vi "Ch_setup_string.vi"(6 "Ch & spans":T1[](array[typedef]) {"low limit (-10V)" format="%.3f"; "high limit (10V)" format="%.3f"}) -> (1 "Output string":string)   [LabVIEW 2013]
uses:
  Controls/Ch_and_Spans.ctl
  Globals/Meas_global.vi
panel:
  out "length":i32
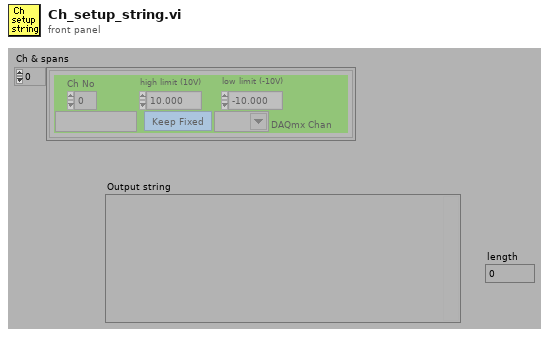
[diagram p1: front panel]
types:
  T1 = typedef "Ch_and_Spans.ctl" = cluster{"high limit (10V)":sgl, "low limit (-10V)":sgl, "Ch No":i16, "Var name":string, "Use Latest Calib":bool, "DAQmx Chan":tag}
  T2 = typedef "Analysis_info_cluster.ctl" = cluster{"Colour":u32, "Inst type":T3, "Inst name":string, "Symbol":string, "Code name":string, "Extra Info":string, "Inst Array":T4, "Extra Titles":string[], "Extra Values":string[], "U":dbl, "u^2":dbl, "u^3":dbl, "u^4":dbl, "Skew_u":dbl, "Kurt_u":dbl, "Sd Error in Mean":dbl, "% u'/U":dbl, "X":dbl, "Y":dbl, "Z":dbl, "Timescale integral to 25%":dbl, "Sd Error in Variance":dbl, "Calib File":path, "Calib Constants":dbl[], "Output Position":bool, "Full Stats":bool, "Av Sampling Rate":dbl, "Av No of Samples":dbl, "Total Meas Time (s)":dbl, "ADAM Ch Name":string}
  T3 = typedef "Inst_type.ctl" = enum16{"Propeller anemometer", "Raw voltage", "Pressure Transducer", "Pitot-static tube", "Preston tube", "Hot wire", "Cross wire 1", "Cross wire 2", "Generic Linear", "Generic Polynomial", "Generic BackPoly", "Fast FID", "Thermocouple", "Cold wire", "Pulsed Wire", "LDA Vel", "LDA Tran time", "LDA Arr time"}
  T4 = typedef "Instrument_Array.ctl" = enum16{"PWA", "LDA", "Analogue"}
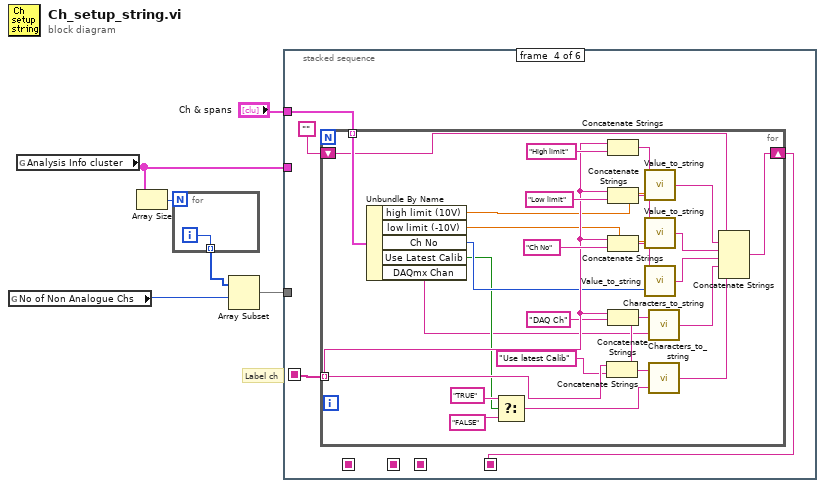
[diagram p0: block diagram]
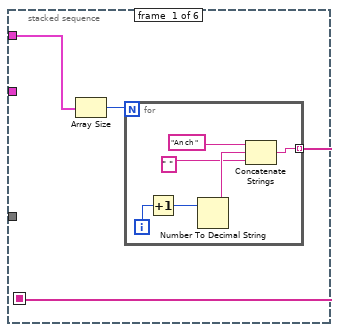
[diagram p2: hidden frame]
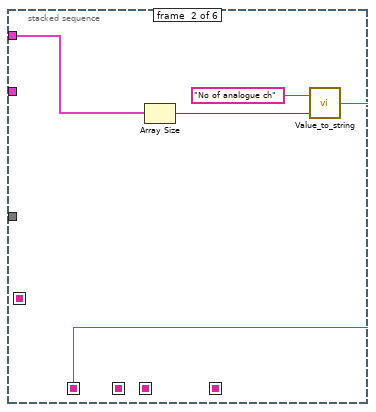
[diagram p3: hidden frame]
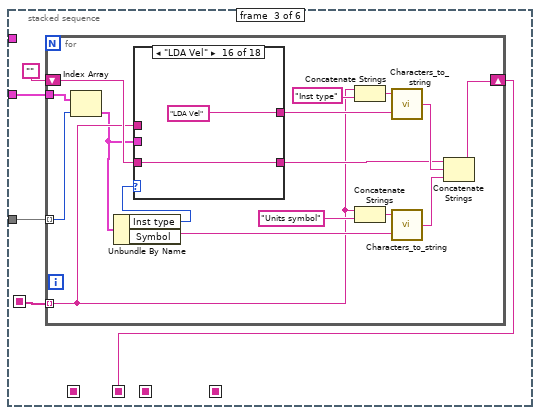
[diagram p4: hidden frame]
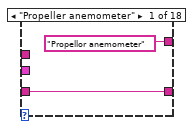
[diagram p5: hidden frame]
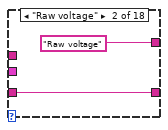
[diagram p6: hidden frame]
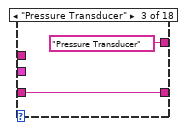
[diagram p7: hidden frame]
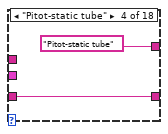
[diagram p8: hidden frame]
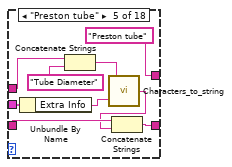
[diagram p9: hidden frame]
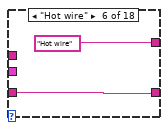
[diagram p10: hidden frame]
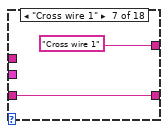
[diagram p11: hidden frame]
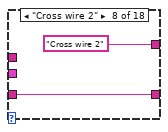
[diagram p12: hidden frame]
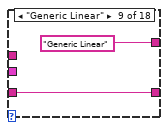
[diagram p13: hidden frame]
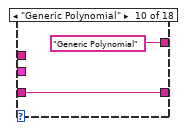
[diagram p14: hidden frame]
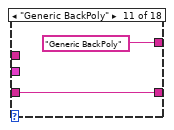
[diagram p15: hidden frame]
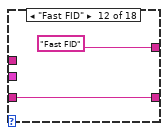
[diagram p16: hidden frame]
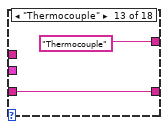
[diagram p17: hidden frame]
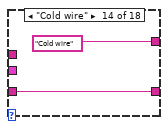
[diagram p18: hidden frame]
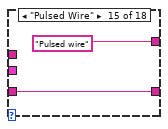
[diagram p19: hidden frame]
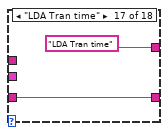
[diagram p20: hidden frame]
diagram:
  # "Label ch"
  n1 = global read "Meas_global.vi" "No of Non Analogue Chs"() -> (w2:i32)
  n2 = global read "Meas_global.vi" "Analysis Info cluster"() -> (w5:T2[])
  n3 = Array Size(array=w5) -> (size(s)=w4:i32)
  n4 = for {
    N: w4 -> [_]
    tunnel: [w7] -> w3 mode=indexing
    i -> [w7]
  }
  n5 = Array Subset(array=w3, index=w2) -> (w1:i32[])  [unwired: 1 in]
  n6 = stacked-sequence {
    seq-local: [_ _ w24 _ _ _] -> [_ _ _ _ _ w136]
    seq-local: [_ _ _ _ w117 _] -> [_ _ _ _ _ w135]
    seq-local: [w9 _ _ _ _ _] -> [_ _ w23 w87 w118 _]
    seq-local: [_ w17 _ _ _ _] -> [_ _ _ _ _ w132]
    seq-local: [_ _ _ w86 _ _] -> [_ _ _ _ _ w131]
    tunnel: "Ch & spans" -> [w8 w18 _ w85 _ _]
    tunnel: w5 -> [_ _ w22 _ w116 _]
    tunnel: w1 -> [_ _ w21 _ w115 _]
    frame #0 {
      n7 = Array Size(array=w8) -> (size(s)=w10:i32)
      n8 = for {
        N: w10 -> [_]
        tunnel: [w12] -> w9 mode=indexing
        i -> [w14]
        n9 = Increment(x=w14) -> (x+1=w13:i32)
        n10 = Number To Decimal String(number=w13) -> (decimal integer string=w16:string)  [unwired: 1 out]
        n11 = Concatenate Strings("An ch ", w16, " ") -> (w12:string)
      }
    }
    frame #1 {
      n12 = Array Size(array=w18) -> (size(s)=w19:i32)
      n13 = call "Value_to_string.vi"("Value"=w19, "Label for value"="No of analogue ch") -> ("Output string"=w17:string)  [unwired: 1 in]
    }
    frame #2 {
      n14 = for {
        shift-right: [w41] -> w24
        shift-left: "" -> [w32]
        tunnel: w23 -> [w29] mode=indexing
        tunnel: w22 -> [w28]
        tunnel: w21 -> [w27] mode=indexing
        n15 = Index Array(array=w28, index=w27) -> (element=w26:T2)
        n16 = Unbundle By Name(w26) -> ("Inst type"=w30:T3, "Symbol"=w40:string)
        n17 = case shown="\"LDA Vel\"" w30 {
          tunnel: ["Propellor anemometer" "Raw voltage" "Pressure Transducer" "Pitot-static tube" "Preston tube" "Hot wire" "Cross wire 1" "Cross wire 2" "Generic Linear" "Generic Polynomial" "Generic BackPoly" "Fast FID" "Thermocouple" "Cold wire" "Pulsed wire" "LDA Vel" "LDA Tran time" "LDA Arr time"] -> w39
          tunnel: w32 -> [w42 w44 w46 w48 w56 w59 w61 w63 w65 w67 w69 w71 w73 w75 w77 w79 w81 w83]
          tunnel: [w42 w44 w46 w48 w55 w59 w61 w63 w65 w67 w69 w71 w73 w75 w77 w79 w81 w83] -> w31
          tunnel: w26 -> [_ _ _ _ w58 _ _ _ _ _ _ _ _ _ _ _ _ _]
          tunnel: w29 -> [_ _ _ _ w51 _ _ _ _ _ _ _ _ _ _ _ _ _]
          frame "Propeller anemometer" {
          }
          frame "Raw voltage" {
          }
          frame "Pressure Transducer" {
          }
          frame "Pitot-static tube" {
          }
          frame "Preston tube" {
            n18 = Unbundle By Name(w58) -> ("Extra Info"=w57:string)
            n19 = Concatenate Strings(w51, "Tube Diameter") -> (w50:string)
            n20 = call "Characters_to_string.vi"("Characters to write"=w57, "Label for characters"=w50) -> ("Output string"=w53:string)
            n21 = Concatenate Strings(w56, w53) -> (w55:string)
          }
          frame "Hot wire" {
          }
          frame "Cross wire 1" {
          }
          frame "Cross wire 2" {
          }
          frame "Generic Linear" {
          }
          frame "Generic Polynomial" {
          }
          frame "Generic BackPoly" {
          }
          frame "Fast FID" {
          }
          frame "Thermocouple" {
          }
          frame "Cold wire" {
          }
          frame "Pulsed Wire" {
          }
          frame "LDA Vel" {
          }
          frame "LDA Tran time" {
          }
          frame "LDA Arr time" {
          }
        }
        n22 = Concatenate Strings(w29, "Inst type") -> (w33:string)
        n23 = Concatenate Strings(w29, "Units symbol") -> (w34:string)
        n24 = call "Characters_to_string.vi"("Characters to write"=w39, "Label for characters"=w33) -> ("Output string"=w35:string)
        n25 = call "Characters_to_string.vi"("Characters to write"=w40, "Label for characters"=w34) -> ("Output string"=w36:string)
        n26 = Concatenate Strings(w31, w35, w36) -> (w41:string)
      }
    }
    frame #3 {
      n27 = for {
        shift-right: [w101] -> w86
        shift-left: "" -> [w89]
        tunnel: w87 -> [w108] mode=indexing
        tunnel: w85 -> [w94] mode=indexing
        n28 = Unbundle By Name(w94) -> ("high limit (10V)"=w99:sgl, "low limit (-10V)"=w98:sgl, "Ch No"=w97:i16, "Use Latest Calib"=w96:bool, "DAQmx Chan"=w95:tag)
        n29 = Select(t="TRUE", s=w96, f="FALSE") -> (s? t:f=w103:string)
        n30 = Concatenate Strings(w108, "Use latest Calib") -> ()  [unwired: 1 out]
        n31 = Concatenate Strings(w108, "High limit") -> (w113:string)
        n32 = Concatenate Strings(w108, "Low limit") -> (w112:string)
        n33 = Concatenate Strings(w108, "Ch No") -> (w109:string)
        n34 = Concatenate Strings(w108, "DAQ Ch") -> (w106:string)
        n35 = call "Value_to_string.vi"("Value"=w99, "Label for value"=w113) -> ("Output string"=w92:string)  [unwired: 1 in]
        n36 = call "Value_to_string.vi"("Value"=w98, "Label for value"=w112) -> ("Output string"=w93:string)  [unwired: 1 in]
        n37 = call "Value_to_string.vi"("Value"=w97, "Label for value"=w109) -> ("Output string"=w91:string)  [unwired: 1 in]
        n38 = call "Characters_to_string.vi"("Characters to write"=w95, "Label for characters"=w106) -> ("Output string"=w100:string)
        n39 = call "Characters_to_string.vi"("Characters to write"=w103, "Label for characters"=w106) -> ("Output string"=w90:string)
        n40 = Concatenate Strings(w89, w92, w93, w91, w100, w90) -> (w101:string)
      }
    }
    frame #4 {
      n41 = for {
        shift-right: [w129] -> w117
        shift-left: "" -> [w130]
        tunnel: w118 -> [w125] mode=indexing
        tunnel: w116 -> [w122]
        tunnel: w115 -> [w121] mode=indexing
        n42 = Index Array(array=w122, index=w121) -> (element=w120:T2)
        n43 = Unbundle By Name(w120) -> ("Calib File"=w123:path)
        n44 = Path To String(path=w123) -> (string=w124:string)
        n45 = Concatenate Strings(w125, "Calib filename") -> (w126:string)
        n46 = call "Characters_to_string.vi"("Characters to write"=w124, "Label for characters"=w126) -> ("Output string"=w127:string)
        n47 = Concatenate Strings(w130, w127) -> (w129:string)
      }
    }
    frame #5 {
      n48 = Concatenate Strings(w132, w136, w135, w131) -> (w133:string)
      "Output string" <- w133
      n49 = String Length(string=w133) -> (length=→"length":i32)
    }
  }
